vi "SearchCommand.vi"() -> ()   [LabVIEW 2009]
panel:
  out "Final Offset":dbl[unit]
  in  "stop":bool
  in  "Step":dbl[unit]
  in  "Start Offset":dbl[unit]
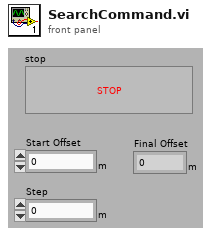
[diagram p1: front panel]
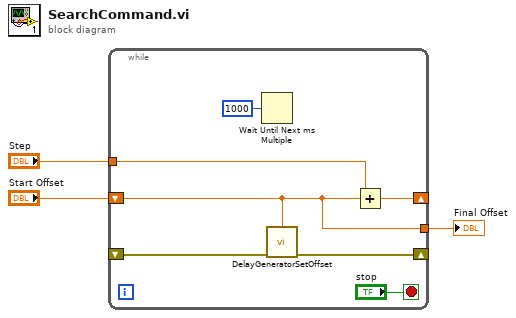
[diagram p0: block diagram]
diagram:
  n1 = while {
    shift-right: [w10] -> _
    shift-left: _ -> [w9]
    shift-right: [w8] -> _
    shift-left: "Start Offset" -> [w4]
    tunnel: "Step" -> [w7]
    tunnel: [w4] -> w1
    stop <- "stop" stop-if-true
    n2 = Wait Until Next ms Multiple(millisecond multiple=u32 1000) -> ()  [unwired: 1 out]
    n3 = call "DelayGeneratorSetOffset.vi"("Offset"=w4, "error in (no error)"=w9) -> ("error out"=w10:errorcluster)  [unwired: 7 in]
    n4 = Add(x=w7, y=w4) -> (x+y=w8:dbl[unit])
  }
  "Final Offset" <- w1
